vi "Create.vi"(5 "HTTPHeaders_NET in":refnum<class "HttpHeaders_NET.lvclass">, 8 "error in (no error)":errorcluster, 11 "NET_HttpHeaders":refnum<k24>) -> (0 "error out":errorcluster, 3 "HTTPHeaders_NET out":refnum<class "HttpHeaders_NET.lvclass">)   [LabVIEW 2018, in "LabVIEWHTTPClient_NET.lvlib" / "HttpHeaders_NET.lvclass"]
uses:
  HttpHeaders_NET.lvclass
  System.Net.Http
  HttpHeaders_NET.lvclass/HttpHeaders_NET.ctl
  Accessors/Write NET_HttpHeaders.vi
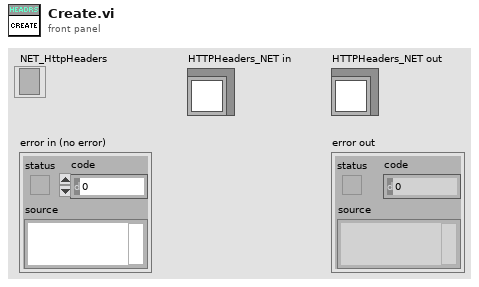
[diagram p1: front panel]
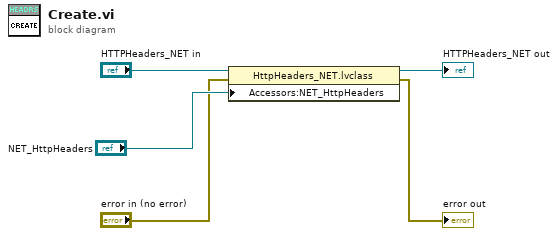
[diagram p0: block diagram]
diagram:
  n1 = property class="HttpHeaders_NET.lvclass"(reference="HTTPHeaders_NET in", error in="error in (no error)", "Accessors:NET_HttpHeaders"="NET_HttpHeaders") -> (reference out=→"HTTPHeaders_NET out":refnum<class "HttpHeaders_NET.lvclass">, error out=→"error out":errorcluster)
